vi "Update Message Routing Info.vi"(0 "message":T1, 5 "receiver host (\"\")":string, 7 "receiver process (\"\")":string, 11 "error in":errorcluster, 12 "source host (\"\")":string, 13 "source process (\"\")":string) -> (4 "message":T1, 15 "error out":errorcluster)   [LabVIEW 2015, in "TLB` Template.lvlib" / "AMC.lvlib"]
doc: "Specifies the routing information for an AMC message.TLB Prime - Application Template 1.3.0.24\nNorm Kirchner, NI Systems Engineering - NI\nCopyright (c) 2014, NI"
uses:
  AMC.lvlib
  Message.ctl
  Tools/Keyed Array/KeyedArray.ctl
  Tools/Keyed Array/Tools_KeyedArray.lvlib
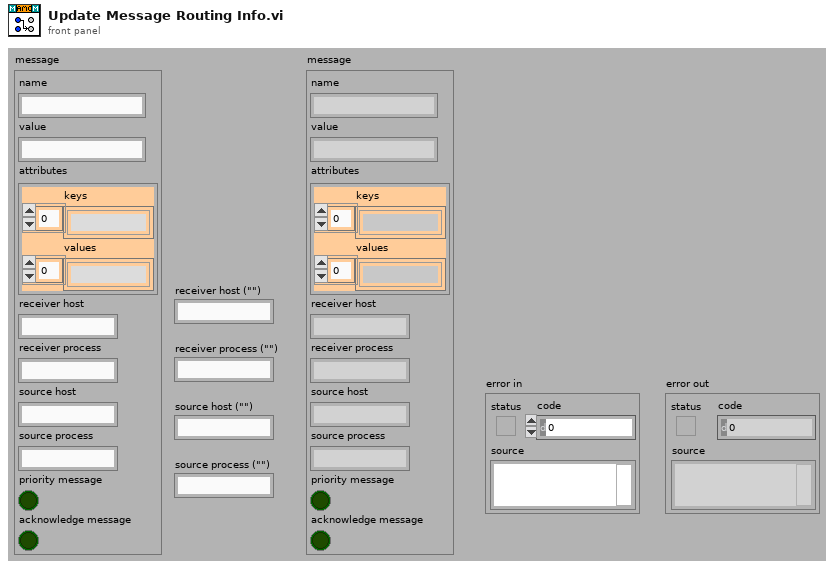
[diagram p1: front panel]
types:
  T1 = typedef "TLB` Template.lvlib/AMC.lvlib/Message.ctl" = cluster{"name":string, "value":string, "attributes":T2, "receiver host":string, "receiver process":string, "source host":string, "source process":string, "priority message":bool, "acknowledge message":bool}
  T2 = typedef "TLB` Template.lvlib/Tools_KeyedArray.lvlib/KeyedArray.ctl" = cluster{"keys":string[], "values":string[]}
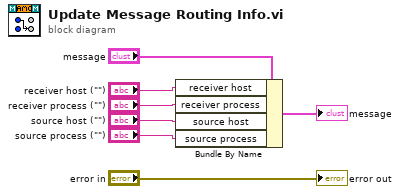
[diagram p0: block diagram]
diagram:
  n1 = Bundle By Name(cluster="message", "receiver host"="receiver host (\"\")", "receiver process"="receiver process (\"\")", "source host"="source host (\"\")", "source process"="source process (\"\")") -> (→"message":T1)
  "error out" <- "error in"
